vi "_Close Communications.vi"(0 "Instrument Channel":string="GPIB/0:4,0", 11 "error in (no error)":errorcluster) -> (15 "error out":errorcluster)   [LabVIEW 2013]
doc: "This VI closes the I/O interface with the instrument."
uses:
  ctl_OperatingMode.ctl
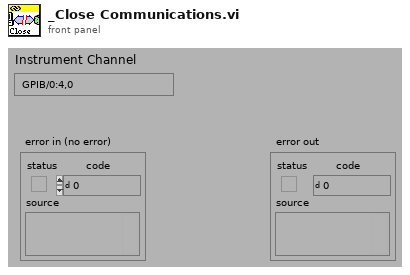
[diagram p1: front panel]
types:
  T1 = typedef "ctl_OperatingMode.ctl" = enum16{"Normal", "Logging", "Simulation w/Zeroes", "Simulation from Log File"}
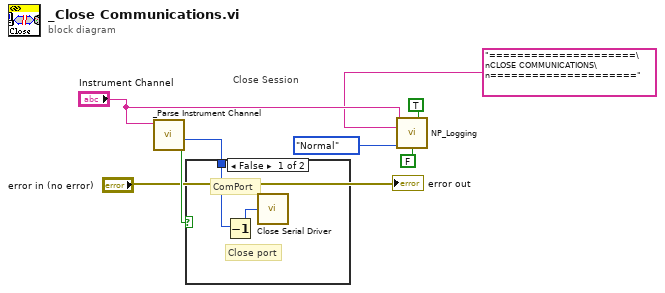
[diagram p0: block diagram]
diagram:
  # "Close Session"
  n1 = call "_Parse Instrument Channel.vi"("Instrument Channel"="Instrument Channel") -> ("T - GPIB, F - RS232"=w7:bool, "Hardware Address"=w8:i32)  [unwired: 6 in, 3 out]
  n2 = case shown="False" w7 {
    tunnel: w8 -> [w9 _]
    frame False {
      # "ComPort"
      # "Close port"
      n3 = Decrement(x=w9) -> (x-1=w10:i32)
      n4 = call <vilib>:"Close Serial Driver.vi"("port number"=w10) -> ()  [unwired: 1 out]
    }
    frame True {
    }
  }
  n5 = call "NP_Logging.vi"("Instrument Channel"="Instrument Channel", "Generic Strings"=TRUE, "String 1 {Write} (in)"="=====================\nCLOSE COMMUNICATIONS\n=====================", "Operating Mode (Logging)"=ctl_OperatingMode."Normal", "String 2 Enable (T)"=FALSE) -> ()  [unwired: 7 in, 4 out]
  "error out" <- "error in (no error)"
